vi "Evaluate Part 2.vi"() -> ()   [LabVIEW 2020]
uses:
  Proto/Group.lvclass
panel:
  out "Array":u64[](array[numeric])
  out "sum 2":u64
  in  "Input":string="#.##..##.\n..#.##.#.\n##......#\n##......#\n..#.##.#.\n..##..##.\n#.#.##.#.\n\n#...##..#\n#....#..#\n..##..###\n#####.##.\n#####.##.\n..##..###\n#....#..#"
  # "10338 too low\n28798 too low"
  # "17385"
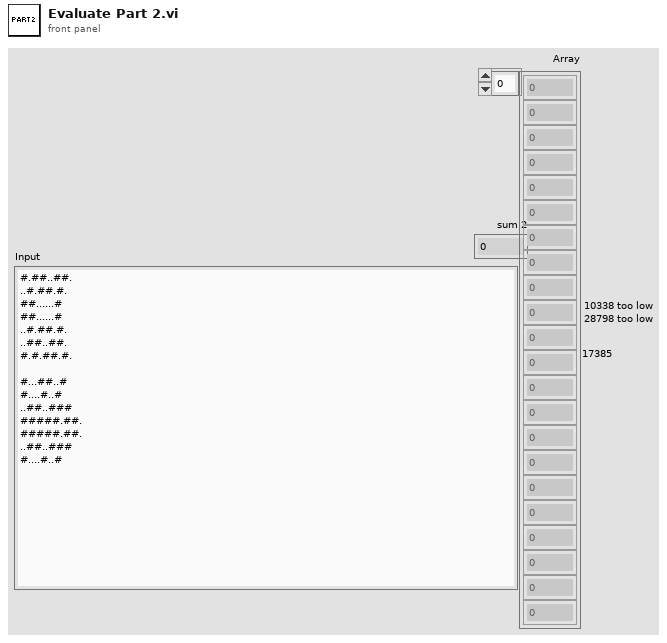
[diagram p1: front panel]
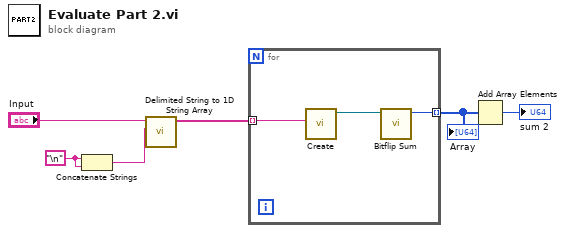
[diagram p0: block diagram]
diagram:
  w3 = "\n"
  n1 = Concatenate Strings(w3, w3) -> (w4:string)
  n2 = call <vilib>:"Delimited String to 1D String Array.vi"("delimiter"=w4, "delimited string"="Input") -> ("string array"=w5:string[])  [unwired: 9 in]
  n3 = for {
    tunnel: w5 -> [w9] mode=indexing
    tunnel: [w7] -> w1 mode=indexing
    n4 = call "Create.vi"("Input"=w9) -> ("Proto"=w8:refnum<class "Group.lvclass">)  [unwired: 9 in, 1 out]
    n5 = call "Bitflip Sum.vi"("Proto in"=w8) -> ("Numeric"=w7:u64)  [unwired: 10 in]
  }
  "Array" <- w1
  n6 = Add Array Elements(numeric array=w1) -> (sum=→"sum 2":u64)
